vi "Do.vi"(8 "error in (no error)":errorcluster, 10 "Actor in":refnum<class "Actor.lvclass">, 11 "Set PID Msg":refnum<class "Set PID Msg.lvclass">) -> (0 "error out":errorcluster, 2 "Actor out":refnum<class "Actor.lvclass">)   [LabVIEW 2021, in "Set PID Msg.lvclass"]
doc: "This VI delivers the message to the actor by calling the appropriate method(s) on the actor."
uses:
  Set PID Msg.lvclass
  Set PID Msg.lvclass/Set PID Msg.ctl
  a0ecedfe-7574-4231-958d-c0a2dd325c31.vi
  Temperature Controller/Temperature Controller.lvclass
  <vilib>/ActorFramework/Actor/Actor.lvclass
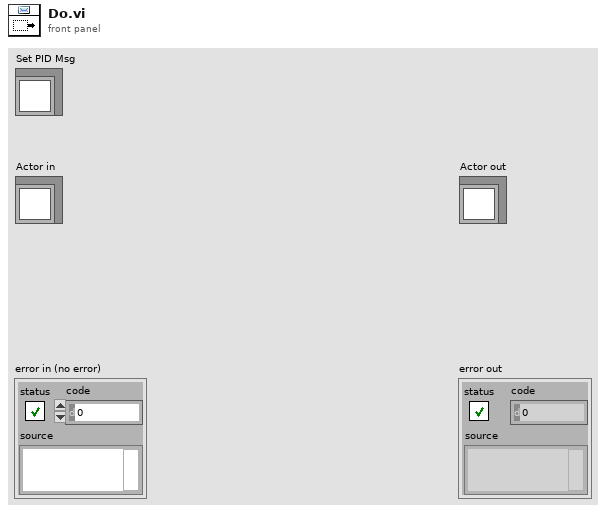
[diagram p1: front panel]
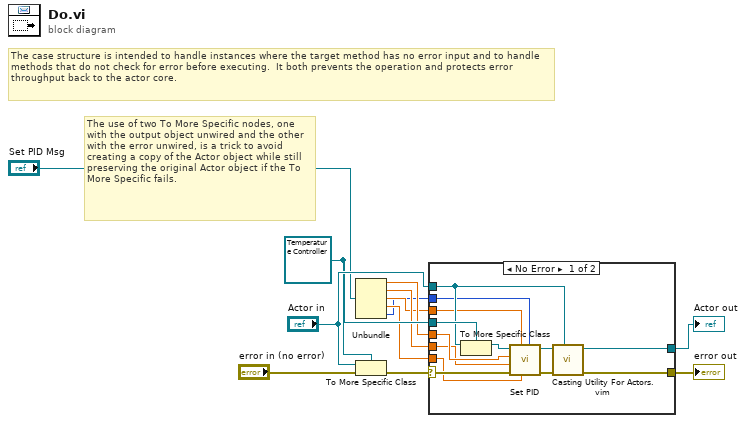
[diagram p0: block diagram]
diagram:
  w7 = refnum<class "Temperature Controller.lvclass"> refnum ("Actor in")
  # "The use of two To More Specific nodes, one with the output object unwired and the other with the error unwired, is a trick to avoid creating a copy of the Actor object while still preserving the original Actor object if the To More Specific fails."
  # "The case structure is intended to handle instances where the target method has no error input and to handle methods that do not check for error before executing.  It both prevents the operation and protects error throughput back to the actor core."
  n1 = Unbundle("Set PID Msg") -> (w5:dbl, w4:dbl, w3:dbl, w2:dbl, w1:i32)
  n2 = To More Specific Class(target class=w7, reference="Actor in", error in="error in (no error)") -> (error out=w6:errorcluster)  [unwired: 1 out]
  n3 = case shown="No Error" w6 {
    selector: w6 -> [w25 w27]
    tunnel: [w19 w27] -> w12
    tunnel: [w20 w26] -> w11
    tunnel: "Actor in" -> [w22 w26]
    tunnel: w7 -> [w23 _]
    tunnel: w5 -> [w17 _]
    tunnel: w4 -> [w16 _]
    tunnel: w3 -> [w15 _]
    tunnel: w2 -> [w14 _]
    tunnel: w1 -> [w13 _]
    frame No Error {
      n4 = To More Specific Class(target class=w23, reference=w22) -> (specific class reference=w24:refnum<class "Temperature Controller.lvclass">)  [unwired: 1 in, 1 out]
      n5 = call-dynamic "Set PID.vi"("Output #"=w13, "D"=w14, "P manual"=w15, "error in (no error)"=w25, "I"=w16, "P"=w17, "Temperature Controller in"=w24) -> ("error out"=w18:errorcluster, "Temperature Controller out"=w21:refnum<class "Temperature Controller.lvclass">)  [unwired: 3 in]
      n6 = call "Casting Utility For Actors.vim"("type"=w22, "error in (no error)"=w18, "Actor in"=w21) -> ("error out"=w19:errorcluster, "Actor out"=w20:refnum<class "Actor.lvclass">)  [unwired: 7 in]
    }
    frame Error {
      # "If type check fails, pass the original object out again."
    }
  }
  "error out" <- w12
  "Actor out" <- w11
